vi "_ReadCalMethod.vi"(4 "Auto-Detect Bias info":T1, 5 "HasESI2":bool, 6 "HasESI1":bool=TRUE, 7 "Method Path":path=path "C:/Users/Public/Molana/Instrument/Project/MS Methods/Automated Calibration Methods/Q1 PPG POS Default.xml") -> (0 "error out":errorcluster, 2 "UseESI1":bool, 3 "GUI Method":T3 {"Mass Ranges"."Res" items=["High/High", "Medium/Medium", "Low/Low", "High/Medium", "High/Low", "Medium/High", "Medium/Low", "Low/High", "Low/Medium"]})   [LabVIEW 2015]
uses:
  Type/_GUI Method.ctl
  Type/_Lens Property.ctl
  Type/_Mass Range Property.ctl
  Type/_Mass Range Parameters.ctl
  Type/_RT Res Type.ctl
  Type/_Run Mode.ctl
  Controls/Auto-Detector Bias Info.ctl
  Controls/Auto-Detector Peak Info.ctl
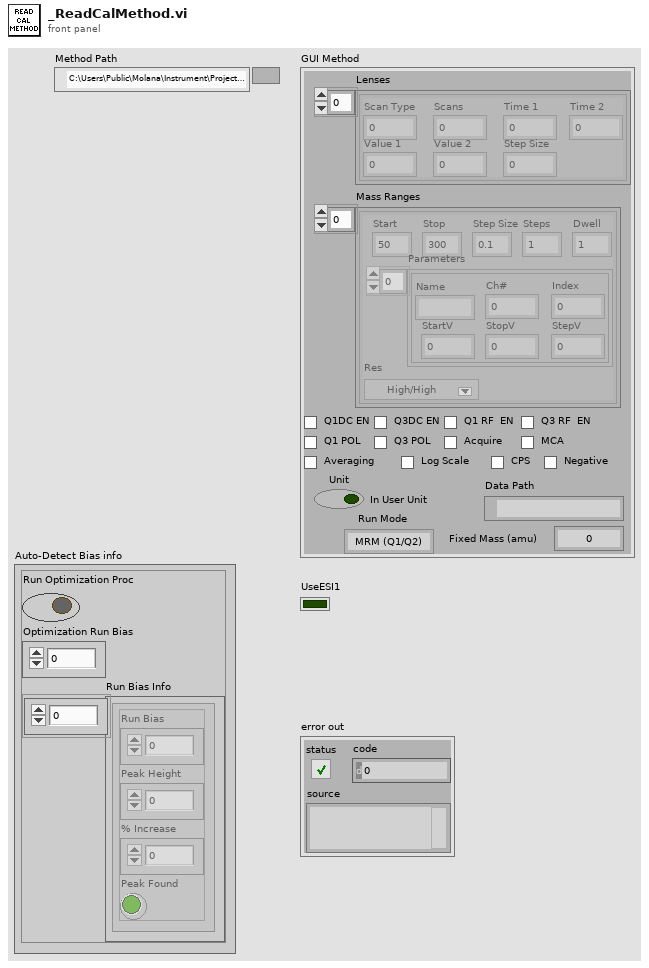
[diagram p1: front panel]
types:
  T1 = typedef "Auto-Detector Bias Info.ctl" = cluster{"Run Optimization Proc":bool, "Optimization Run Bias":u32, "Run Bias Info":T2[]}
  T2 = typedef "Auto-Detector Peak Info.ctl" = cluster{"Run Bias":u32, "Peak Height":dbl, "% Increase":dbl, "Peak Found":bool}
  T3 = typedef "_GUI Method.ctl" = cluster{"Lenses":T4[], "Mass Ranges":T5[], "Acquire":bool, "MCA":bool, "Q1DC EN":bool, "Q1 POL":bool, "Q3 POL":bool, "Q1 RF  EN":bool, "Averaging":bool, "Log Scale":bool, "CPS":bool, "Unit":bool, "Data Path":path, "Run Mode":T8, "Fixed Mass (amu)":dbl, "Q3DC EN":bool, "Q3 RF  EN":bool, "Negative":bool}
  T4 = typedef "_Lens Property.ctl" = cluster{"Scan Type":u8, "Scans":i32, "Time 1":dbl, "Time 2":dbl, "Value 1":dbl, "Value 2":dbl, "Step Size":dbl}
  T5 = typedef "_Mass Range Property.ctl" = cluster{"Start":dbl, "Stop":dbl, "Step Size":dbl, "Steps":i32, "Dwell":dbl, "Parameters":T6[], "Res":T7}
  T6 = typedef "_Mass Range Parameters.ctl" = cluster{"Name":string, "Ch#":u8, "StartV":dbl, "StopV":dbl, "StepV":dbl, "Index":u8}
  T7 = typedef "_RT Res Type.ctl" = u16
  T8 = typedef "_Run Mode.ctl" = enum16{"MRM (Q1/Q2)", "Q1 Scan", "Q1 SRM", "Q2 Scan", "Q2 SRM", "Product Scan", "Precursor Scan", "Neutral Loss", "Neutral Gain"}
  T9 = cluster{"ExptLevelParameters":string[][], "MassRanges":string[][], " MRParameters":T6[][]}
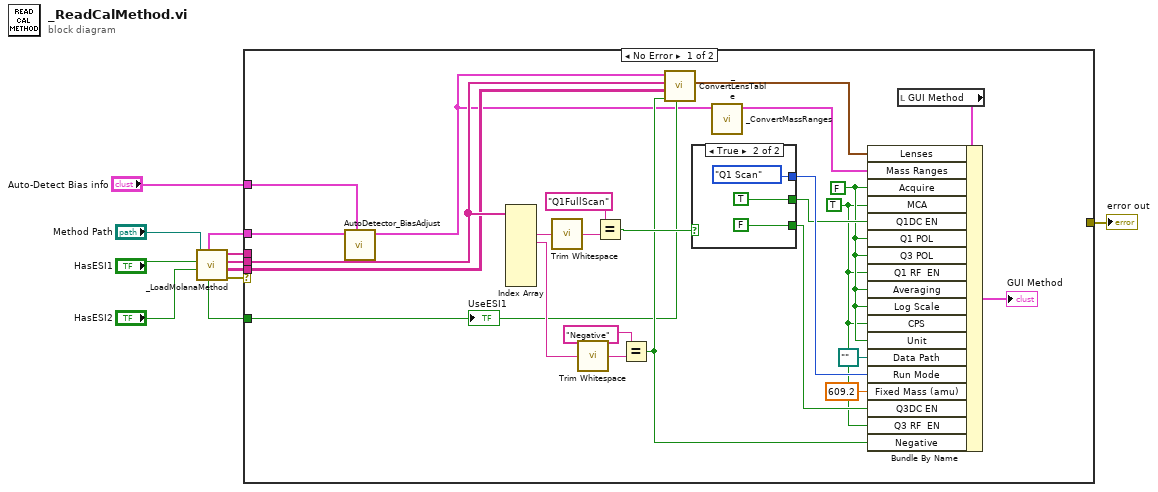
[diagram p0: block diagram]
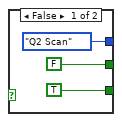
[diagram p2: hidden frame]
diagram:
  n1 = call "_LoadMolanaMethod.vi"("HasESI2"="HasESI2", "HasESI1"="HasESI1", "Path"="Method Path") -> ("error out"=w9:errorcluster, "MethodLevelParameters"=w4:string[][], "Expt"=w3:string[], "Method"=w2:string[], "UseESI1"=w6:bool, "ExptParamAndMR"=w5:T9)  [unwired: 1 in]
  n2 = case shown="No Error" w9 {
    selector: w9 -> [_ w43]
    tunnel: [_ w43] -> w11
    tunnel: w6 -> [w15 _]
    tunnel: w5 -> [w14 _]
    tunnel: w4 -> [w16 _]
    tunnel: w3 -> [w17 _]
    tunnel: w2 -> [_ _]
    tunnel: "Auto-Detect Bias info" -> [w12 _]
    frame No Error {
      w21 = TRUE ("MCA")
      w25 = FALSE
      n3 = call "AutoDetector_BiasAdjust.vi"("Auto-Detect Bias info"=w12, "ExptParamAndMR"=w14) -> ("ExptParamAndMR"=w13:T9)  [unwired: 9 in]
      n4 = Index Array(array=w17) -> (element #2=w35:string, element #3=w26:string)  [unwired: 8 in, 6 out]
      n5 = call <vilib>:"Trim Whitespace.vi"("string"=w35) -> ("trimmed string"=w34:string)  [unwired: 1 in]
      n6 = call <vilib>:"Trim Whitespace.vi"("string"=w26) -> ("trimmed string"=w27:string)  [unwired: 1 in]
      n7 = Equal?(x="Q1FullScan", y=w34) -> (x = y?=w32:bool)
      n8 = Equal?(x="Negative", y=w27) -> (x = y?=w20:bool)
      n9 = call "_ConvertLensTable.vi"("UseESI1"=w15, "IsNegative"=w20, "MethodLevelParameters"=w16, "Expt"=w17, "ExptParamAndMR"=w13) -> ("LensTable"=w19:T4[])  [unwired: 3 in]
      n10 = case shown="True" w32 {
        tunnel: [_Run_Mode."Q2 Scan" ("Run Mode") _Run_Mode."Q1 Scan" ("Run Mode")] -> w31
        tunnel: [FALSE TRUE] -> w30
        tunnel: [TRUE FALSE] -> w29
        frame False {
        }
        frame True {
        }
      }
      n11 = call "_ConvertMassRanges.vi"("ExptParamAndMR"=w13) -> ("MassRanges"=w18:T5[])  [unwired: 6 in]
      n12 = local read "GUI Method"() -> (w36:T3)
      n13 = Bundle By Name(cluster=w36, "Lenses"=w19, "Mass Ranges"=w18, "Acquire"=w25, "MCA"=w21, "Q1DC EN"=w30, "Q1 POL"=w25, "Q3 POL"=w25, "Q1 RF  EN"=w21, "Averaging"=w25, "Log Scale"=w25, "CPS"=w21, "Unit"=w25, "Data Path"=path "", "Run Mode"=w31, "Fixed Mass (amu)"=609.2, "Q3DC EN"=w29, "Q3 RF  EN"=w21, "Negative"=w20) -> (→"GUI Method":T3)
      "UseESI1" <- w15
    }
    frame Error {
      # "Failed to load the method or the method is invalid"
    }
  }
  "error out" <- w11
